vi "spike_data_packete_1.vi"(8 "Log File in":refnum<k34>, 11 "data out":string) -> (3 "output cluster":T1)   [LabVIEW 2017]
uses:
  UI Error Handlers/support/Logging/Control 2.ctl
  Globals/Global - Configuration Options.vi
panel:
  out "data":string
  out "error out":errorcluster
  out "BR3_3 (bending X) 4":i16
  out "data  2":string
  out "SYNC 2":string
  out "BR3_4 (bending X) 4":i16
  out "BR2_4 (torsion) 4":i16
  out "BR1_4 (axial_force_ 4":i16
  out "BR4_7 (bending Y) 7":i16
  out "BR3_7 (bending X) 7":i16
  out "BR2_7 (torsion)6 2":i16
  out "BR1_7 (axial_force_ 7":i16
  out "BR4_6 (bending Y) 6":i16
  out "BR3_6 (bending X) 6":i16
  out "BR2_6 (torsion)6":i16
  out "BR1_6 (axial_force_ 6":i16
  out "BR4_5 (bending Y) 5":i16
  out "BR3_5 (bending X) 5":i16
  out "BR2_5 (torsion) 5":i16
  out "BR1_5 (axial_force_ 5":i16
  out "BR4_4 (bending Y) 4":i16
  out "BR4_3 (bending Y) 3":i16
  out "BR2_3 (torsion) 3":i16
  out "BR1_3 (axial_force_ 3":i16
  out "BR4_2 (bending Y) 2":i16
  out "BR3_2 (bending X) 2":i16
  out "BR2_2 (torsion) 2":i16
  out "BR1_2 (axial_force_ 2":i16
  out "BR4_1 (bending Y)":i16
  out "BR3_1 (bending X)":i16
  out "BR2_1 (torsion)":i16
  out "BR1_1 (axial_force)":i16
  out "SPER":i16
  out "SPEF":i8
  out "RSSI":i16
  out "PKT":i16
  out "DIN":i8
  out "CMD":i8
  out "DEV":i8
  out "RES":i8
  out "LEN":i8
  out "SYN":i16
  in  "?":T1
  out "DIN":string
  out "DEV":string
  out "RES":string
  out "LEN":string
  out "SYNC":string
  out "CMD":string
  out "Received Data 4":dbl[](graph)
  out "BR4_5 (bending Y) 5":string
  out "BR3_5 (bending X) 5":string
  out "BR4_7 (bending Y) 7":string
  out "BR3_7 (bending X) 7":string
  out "BR2_7 (torsion)6 2":string
  out "BR1_7 (axial_force_ 7":string
  out "BR4_6 (bending Y) 6":string
  out "BR3_6 (bending X) 6":string
  out "BR2_6 (torsion)6":string
  out "BR1_6 (axial_force_ 6":string
  out "BR2_5 (torsion) 5":string
  out "BR1_5 (axial_force_ 5":string
  out "BR4_4 (bending Y) 4":string
  out "BR3_4 (bending X) 4":string
  out "BR2_4 (torsion) 4":string
  out "BR1_4 (axial_force_ 4":string
  out "BR4_3 (bending Y) 3":string
  out "BR3_3 (bending X) 3":string
  out "BR2_3 (torsion) 3":string
  out "BR1_3 (axial_force_ 3":string
  out "BR4_2 (bending Y) 2":string
  out "BR3_2 (bending X) 2":string
  out "RSSI":string
  out "PKT":string
  out "SPEF":string
  out "SPER":string
  out "BR2_2 (torsion) 2":string
  out "BR1_2 (axial_force_ 2":string
  out "BR4_1 (bending Y)":string
  out "BR3_1 (bending X)":string
  out "BR2_1 (torsion)":string
  out "BR1_1 (axial_force_":string
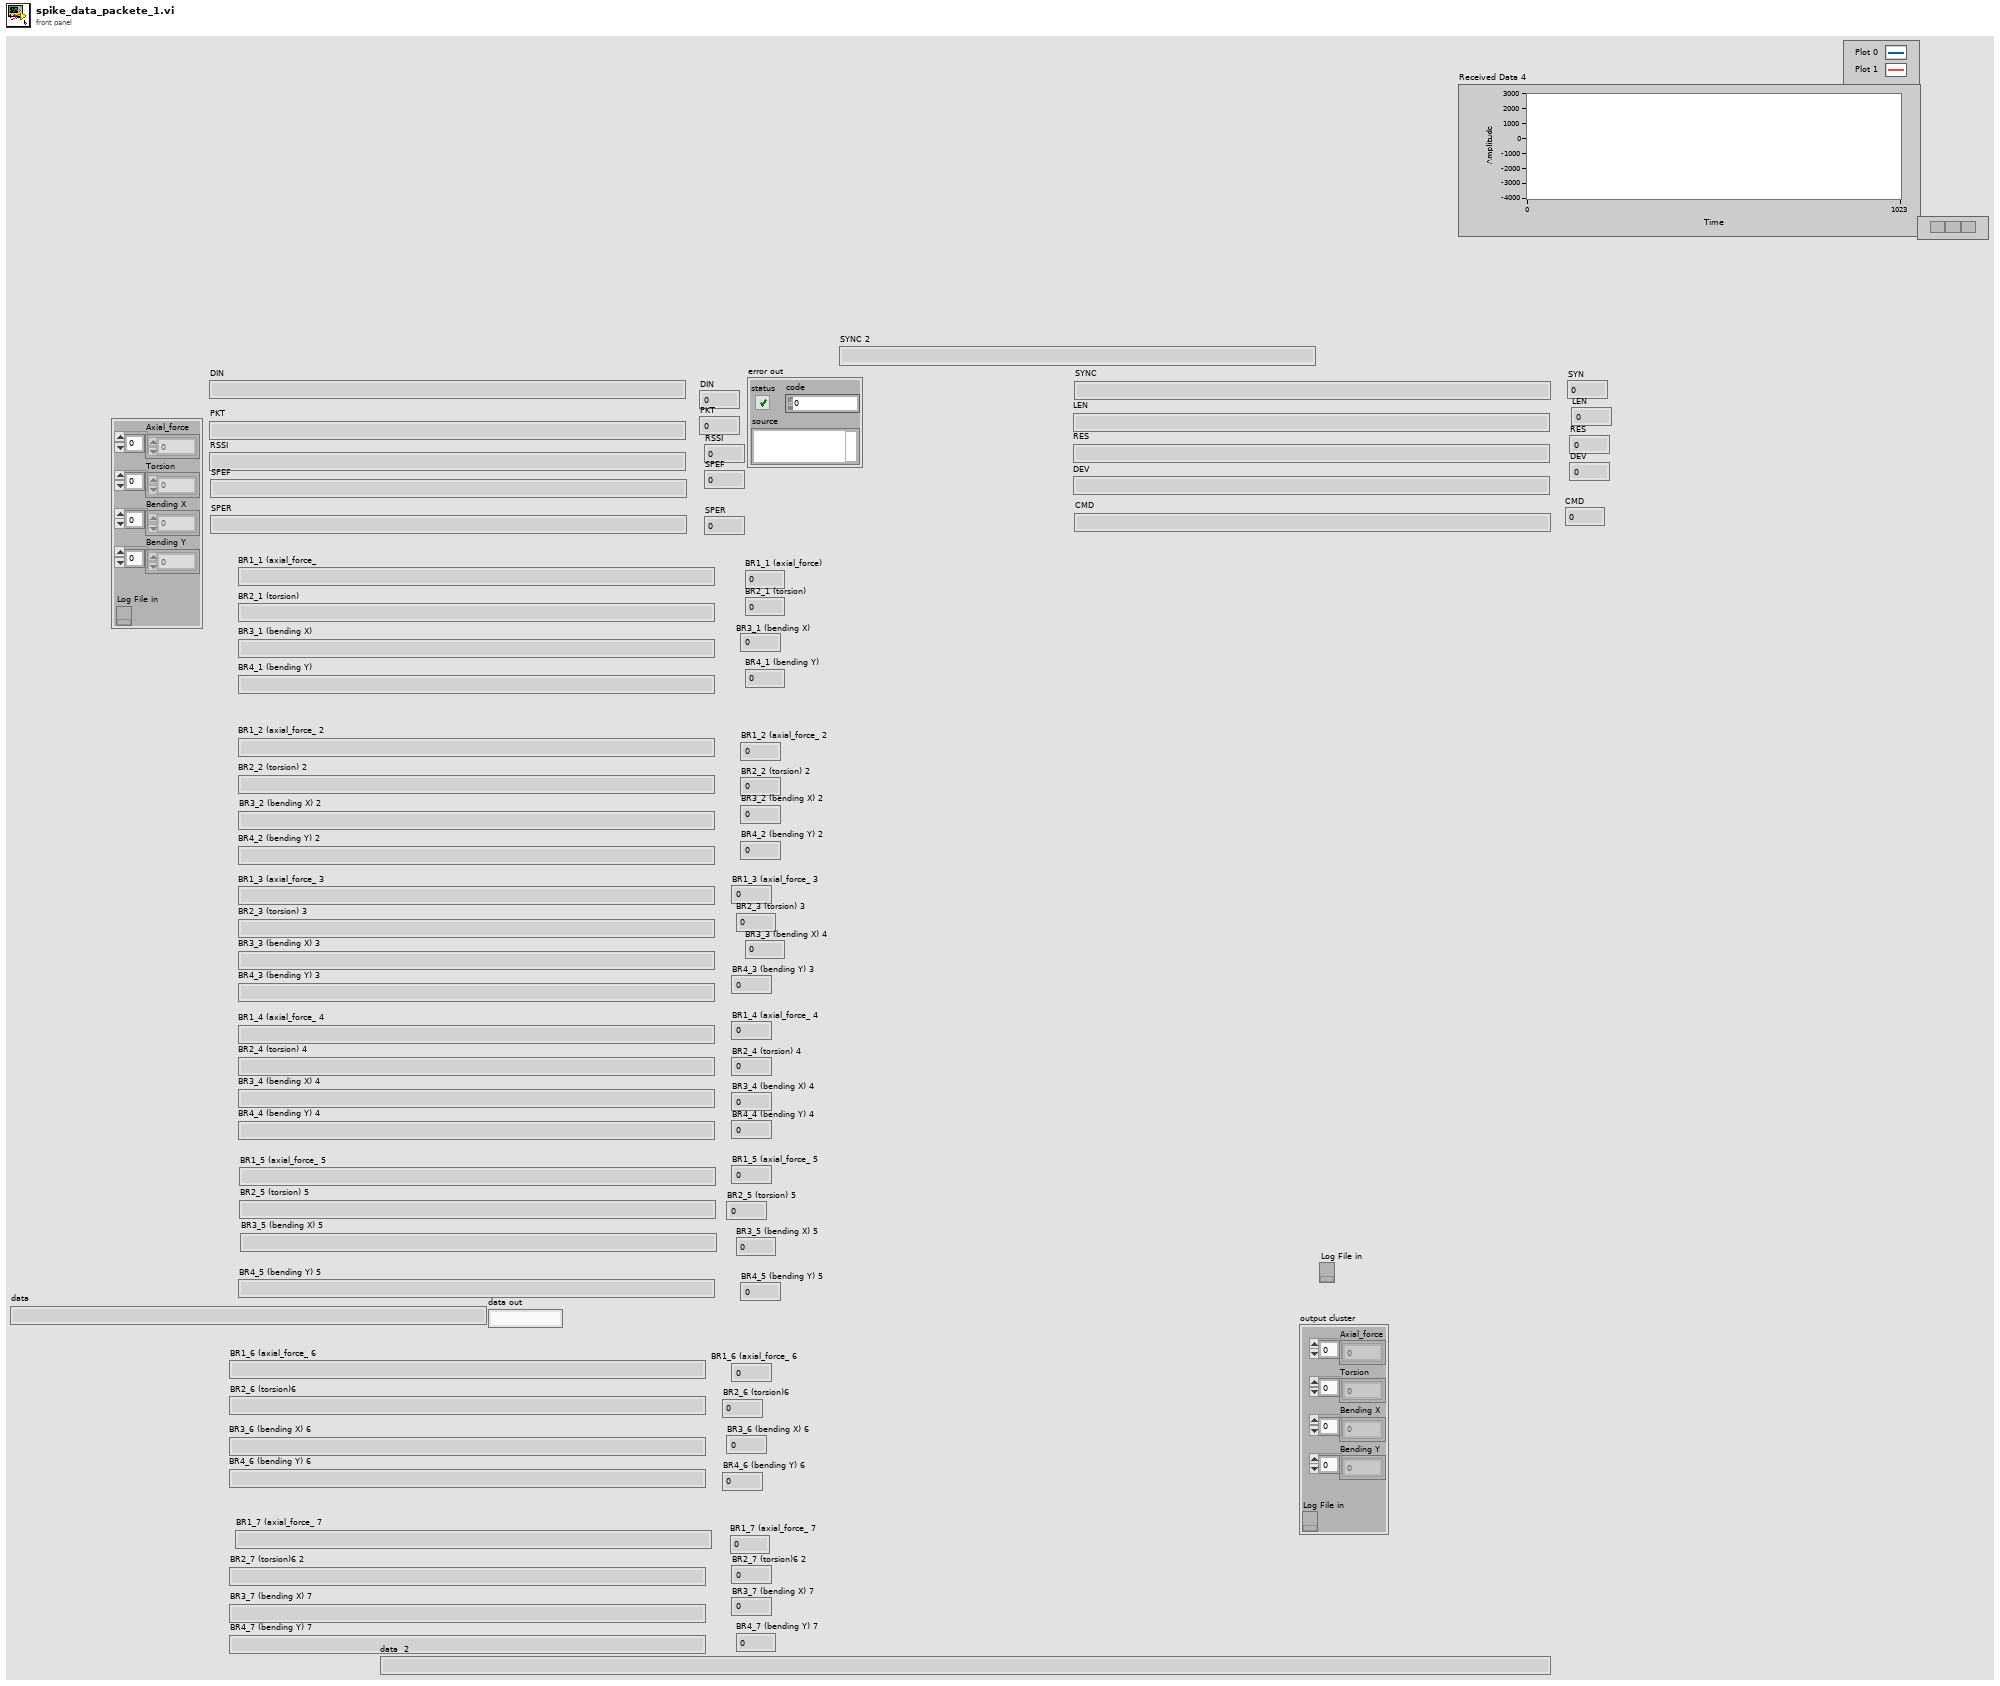
[diagram p1: front panel]
types:
  T1 = typedef "Control 2.ctl" = cluster{"Axial_force":i16[], "Torsion":i16[], "Bending X":i16[], "Bending Y":i16[], "Log File in":refnum<k34>}
  T2 = cluster{"A(I16) 11":i16, "A(I16) 12":i16, "A(I16) 13":i16}
  T3 = cluster{"A(I16) 11":i16, "A(I16) 12":i16, "A(I16) 13":i16, "A(I16) 14":i16, "A(I16) 15":i16, "A(I16) 16":i16, "A(I16) 17":i16}
  T4 = enum16{"big-endian, network order", "native, host order", "little-endian"}
  T5 = cluster{"A(I16)":i16, "A(I8) 2":i8, "A(I8) 3":i8, "A(I18) 4":i8, "A(I8) 5":i8, "A(I8) 6":i8, "A(I16) 7":i16, "A(I8) 8":i8, "A(I8) 9":i8, "A(I16) 10":i16, "A(I16) 11":i16, "A(I16) 12":i16, "A(I16) 13":i16, "A(I16) 14":i16, "A(I16) 15":i16, "A(I16) 16":i16, "A(I16) 17":i16, "A(I16) 18":i16, "A(I16) 19":i16, "A(I16) 20":i16, "A(I16) 21":i16, "A(I16) 22":i16, "A(I16) 23":i16, "A(I16) 24":i16, "A(I16) 25":i16, "A(I16) 26":i16, "A(I16) 27":i16, "A(I16) 28":i16, "A(I16) 29":i16, "A(I16) 30":i16, "A(I16) 31":i16, "A(I16) 32":i16, "A(I16) 33":i16, "A(I16) 34":i16, "A(I16) 35":i16, "A(I16) 36":i16, "A(I16) 37":i16, "A(I16) 38":i16, "A(I16) 39":i16, "A(I16) 40":i16, "A(I16) 41":i16, "A(I16) 42":i16, "A(I16) 43":i16, "A(I16) 44":i16, "A(I16) 45":i16, "A(I16) 46":i16, "A(I16) 47":i16, "A(I16) 48":i16, "A(I16) 49":i16, "A(I16) 50":i16, "A(I16) 51":i16, "A(I16) 52":i16, "A(I16) 53":i16, "A(I16) 54":i16, "A(I16) 55":i16, "A(I16) 56":i16, "A(I16) 57":i16, "A(I16) 58":i16, "A(I16) 59":i16, "A(I16) 60":i16, "A(I16) 61":i16, "A(I16) 62":i16, "A(I16) 63":i16, "A(I16) 64":i16, "A(I16) 65":i16, "A(I16) 66":i16, "A(I16) 67":i16, "A(I16) 68":i16, "A(I16) 69":i16, "A(I16) 70":i16}
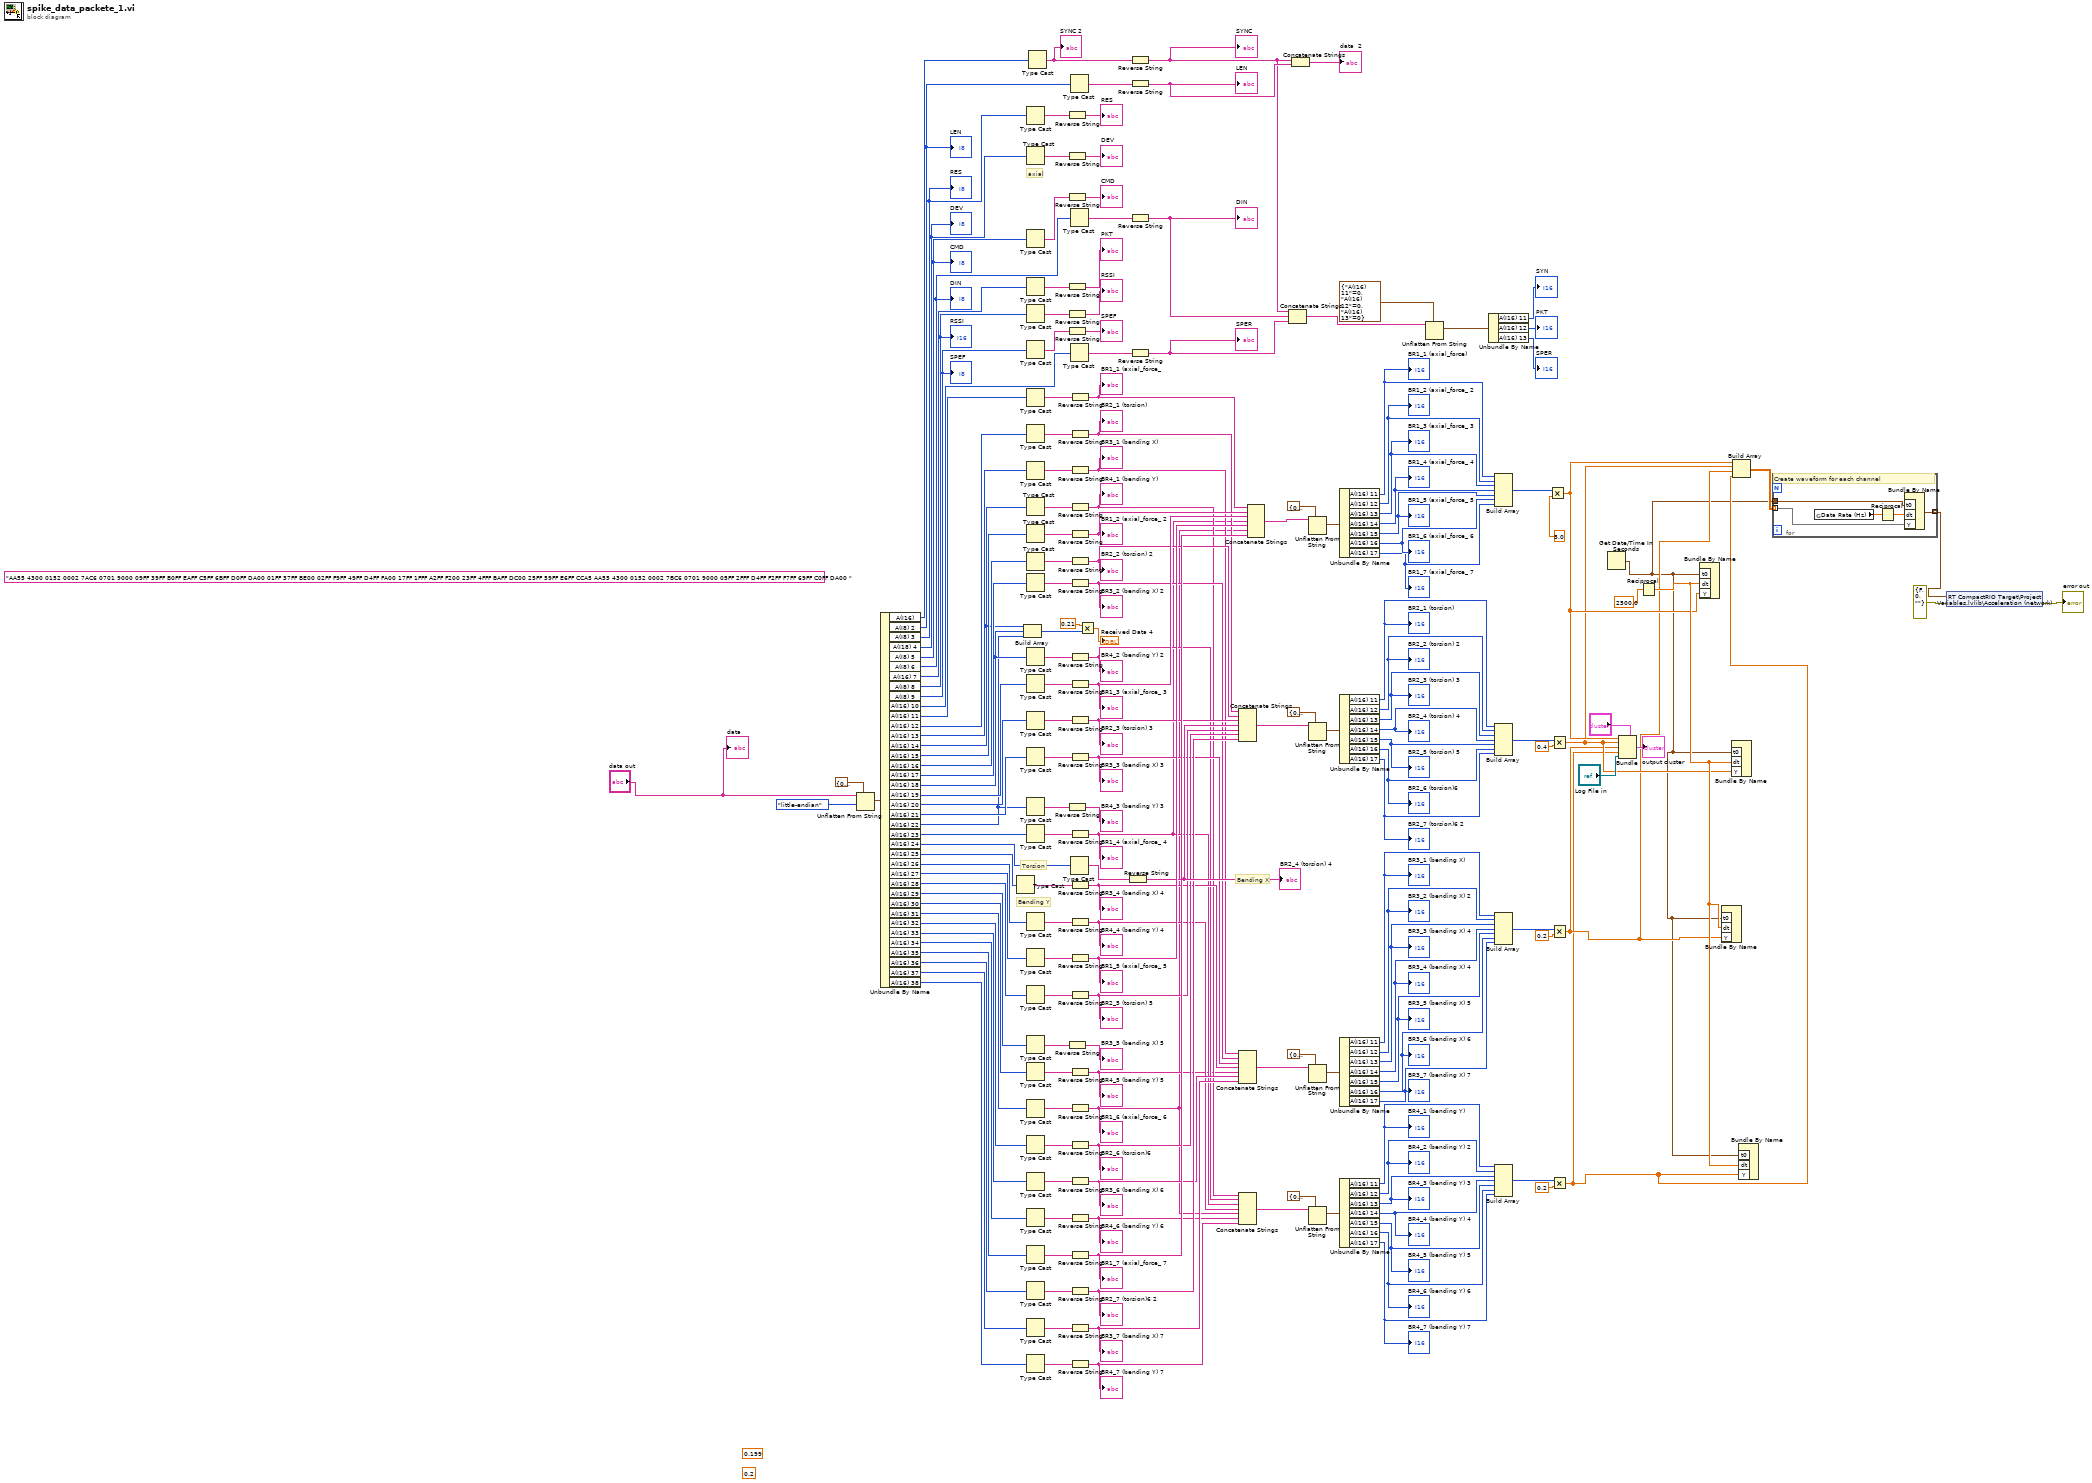
[diagram p0: block diagram]
diagram:
  (unwired) "AA55 4300 0152 0002 7AC6 0701 9000 09FF 39FF B0FF EAFF C5FF 6BFF D0FF DA00 01FF 37FF BE00 02FF F9FF 49FF D4FF FA00 17FF 1FFF A2FF F200 23FF 4FFF BAFF DC00 25FF 59FF E6FF CCA5 AA55 4300 0152 0002 7BC6 0701 9000 05FF 2FFF D4FF F2FF F7FF 69FF C0FF DA00 " ("data")
  (unwired) 0.2
  (unwired) 0.199
  # "Bending Y"
  # "Bending X"
  # "axial"
  # "Torsion"
  n1 = Unflatten From String(type=T5 {"A(I16)"=0, "A(I8) 2"=0, "A(I8) 3"=0, "A(I18) 4"=0, "A(I8) 5"=0, "A(I8) 6"=0, "A(I16) 7"=0, "A(I8) 8"=0, "A(I8) 9"=0, "A(I16) 10"=0, "A(I16) 11"=0, "A(I16) 12"=0, "A(I16) 13"=0, "A(I16) 14"=0, "A(I16) 15"=0, "A(I16) 16"=0, "A(I16) 17"=0, "A(I16) 18"=0, "A(I16) 19"=0, "A(I16) 20"=0, "A(I16) 21"=0, "A(I16) 22"=0, "A(I16) 23"=0, "A(I16) 24"=0, "A(I16) 25"=0, "A(I16) 26"=0, "A(I16) 27"=0, "A(I16) 28"=0, "A(I16) 29"=0, "A(I16) 30"=0, "A(I16) 31"=0, "A(I16) 32"=0, "A(I16) 33"=0, "A(I16) 34"=0, "A(I16) 35"=0, "A(I16) 36"=0, "A(I16) 37"=0, "A(I16) 38"=0, "A(I16) 39"=0, "A(I16) 40"=0, "A(I16) 41"=0, "A(I16) 42"=0, "A(I16) 43"=0, "A(I16) 44"=0, "A(I16) 45"=0, "A(I16) 46"=0, "A(I16) 47"=0, "A(I16) 48"=0, "A(I16) 49"=0, "A(I16) 50"=0, "A(I16) 51"=0, "A(I16) 52"=0, "A(I16) 53"=0, "A(I16) 54"=0, "A(I16) 55"=0, "A(I16) 56"=0, "A(I16) 57"=0, "A(I16) 58"=0, "A(I16) 59"=0, "A(I16) 60"=0, "A(I16) 61"=0, "A(I16) 62"=0, "A(I16) 63"=0, "A(I16) 64"=0, "A(I16) 65"=0, "A(I16) 66"=0, "A(I16) 67"=0, "A(I16) 68"=0, "A(I16) 69"=0, "A(I16) 70"=0}, binary string="data out", byte order (0:big-endian, network order)=T4."little-endian") -> (value=w148:T5)  [unwired: 2 in, 2 out]
  n2 = Unbundle By Name(w148) -> ("A(I16)"=w140:i16, "A(I8) 2"=w139:i8, "A(I8) 3"=w138:i8, "A(I18) 4"=w133:i8, "A(I8) 5"=w132:i8, "A(I8) 6"=w131:i8, "A(I16) 7"=w130:i16, "A(I8) 8"=w129:i8, "A(I8) 9"=w128:i8, "A(I16) 10"=w127:i16, "A(I16) 11"=w101:i16, "A(I16) 12"=w64:i16, "A(I16) 13"=w63:i16, "A(I16) 14"=w104:i16, "A(I16) 15"=w126:i16, "A(I16) 16"=w118:i16, "A(I16) 17"=w114:i16, "A(I16) 18"=w110:i16, "A(I16) 19"=w125:i16, "A(I16) 20"=w120:i16, "A(I16) 21"=w75:i16, "A(I16) 22"=w58:i16, "A(I16) 23"=w124:i16, "A(I16) 24"=w119:i16, "A(I16) 25"=w57:i16, "A(I16) 26"=w109:i16, "A(I16) 27"=w123:i16, "A(I16) 28"=w117:i16, "A(I16) 29"=w113:i16, "A(I16) 30"=w108:i16, "A(I16) 31"=w122:i16, "A(I16) 32"=w115:i16, "A(I16) 33"=w112:i16, "A(I16) 34"=w107:i16, "A(I16) 35"=w121:i16, "A(I16) 36"=w116:i16, "A(I16) 37"=w111:i16, "A(I16) 38"=w106:i16)
  "LEN" <- w139
  "RES" <- w138
  "DEV" <- w133
  "CMD" <- w132
  "DIN" <- w131
  "RSSI" <- w129
  "SPEF" <- w128
  n3 = Type Cast(x=w57) -> (*(type *) &x=w167:string)  [unwired: 1 in]
  n4 = Build Array(w104, w110, w58) -> (w150:i16[])
  n5 = Type Cast(x=w138) -> (*(type *) &x=w146:string)  [unwired: 1 in]
  n6 = Type Cast(x=w133) -> (*(type *) &x=w145:string)  [unwired: 1 in]
  n7 = Type Cast(x=w132) -> (*(type *) &x=w144:string)  [unwired: 1 in]
  n8 = Type Cast(x=w130) -> (*(type *) &x=w188:string)  [unwired: 1 in]
  n9 = Type Cast(x=w129) -> (*(type *) &x=w187:string)  [unwired: 1 in]
  n10 = Type Cast(x=w128) -> (*(type *) &x=w184:string)  [unwired: 1 in]
  n11 = Type Cast(x=w101) -> (*(type *) &x=w186:string)  [unwired: 1 in]
  n12 = Type Cast(x=w64) -> (*(type *) &x=w183:string)  [unwired: 1 in]
  n13 = Type Cast(x=w63) -> (*(type *) &x=w182:string)  [unwired: 1 in]
  n14 = Type Cast(x=w104) -> (*(type *) &x=w181:string)  [unwired: 1 in]
  n15 = Type Cast(x=w126) -> (*(type *) &x=w180:string)  [unwired: 1 in]
  n16 = Type Cast(x=w118) -> (*(type *) &x=w179:string)  [unwired: 1 in]
  n17 = Type Cast(x=w114) -> (*(type *) &x=w174:string)  [unwired: 1 in]
  n18 = Type Cast(x=w110) -> (*(type *) &x=w175:string)  [unwired: 1 in]
  n19 = Type Cast(x=w125) -> (*(type *) &x=w173:string)  [unwired: 1 in]
  n20 = Type Cast(x=w120) -> (*(type *) &x=w172:string)  [unwired: 1 in]
  n21 = Type Cast(x=w75) -> (*(type *) &x=w171:string)  [unwired: 1 in]
  n22 = Type Cast(x=w58) -> (*(type *) &x=w170:string)  [unwired: 1 in]
  n23 = Type Cast(x=w124) -> (*(type *) &x=w165:string)  [unwired: 1 in]
  n24 = Type Cast(x=w109) -> (*(type *) &x=w168:string)  [unwired: 1 in]
  n25 = Type Cast(x=w123) -> (*(type *) &x=w164:string)  [unwired: 1 in]
  n26 = Type Cast(x=w117) -> (*(type *) &x=w163:string)  [unwired: 1 in]
  n27 = Type Cast(x=w113) -> (*(type *) &x=w154:string)  [unwired: 1 in]
  n28 = Type Cast(x=w108) -> (*(type *) &x=w152:string)  [unwired: 1 in]
  n29 = Type Cast(x=w122) -> (*(type *) &x=w162:string)  [unwired: 1 in]
  n30 = Type Cast(x=w115) -> (*(type *) &x=w159:string)  [unwired: 1 in]
  n31 = Type Cast(x=w112) -> (*(type *) &x=w161:string)  [unwired: 1 in]
  n32 = Type Cast(x=w107) -> (*(type *) &x=w160:string)  [unwired: 1 in]
  n33 = Type Cast(x=w121) -> (*(type *) &x=w155:string)  [unwired: 1 in]
  n34 = Type Cast(x=w116) -> (*(type *) &x=w158:string)  [unwired: 1 in]
  n35 = Type Cast(x=w111) -> (*(type *) &x=w156:string)  [unwired: 1 in]
  n36 = Type Cast(x=w106) -> (*(type *) &x=w157:string)  [unwired: 1 in]
  n37 = Type Cast(x=w140) -> (*(type *) &x=w105:string)  [unwired: 1 in]
  "SYNC 2" <- w105
  n38 = Reverse String(1:w146) -> (0:→"RES":string)
  n39 = Reverse String(1:w145) -> (0:→"DEV":string)
  n40 = Reverse String(1:w144) -> (0:→"CMD":string)
  n41 = Reverse String(1:w188) -> (0:→"PKT":string)
  n42 = Reverse String(1:w187) -> (0:→"RSSI":string)
  n43 = Reverse String(1:w184) -> (0:→"SPEF":string)
  n44 = Reverse String(1:w170) -> (0:→"BR4_3 (bending Y) 3":string)
  n45 = Reverse String(1:w154) -> (0:→"BR3_5 (bending X) 5":string)
  n46 = Type Cast(x=w139) -> (*(type *) &x=w147:string)  [unwired: 1 in]
  n47 = Type Cast(x=w131) -> (*(type *) &x=w137:string)  [unwired: 1 in]
  n48 = Type Cast(x=w127) -> (*(type *) &x=w185:string)  [unwired: 1 in]
  n49 = Type Cast(x=w119) -> (*(type *) &x=w166:string)  [unwired: 1 in]
  n50 = Reverse String(1:w186) -> (0:w13:string)
  "BR1_1 (axial_force_" <- w13
  n51 = Reverse String(1:w183) -> (0:w83:string)
  "BR2_1 (torsion)" <- w83
  n52 = Reverse String(1:w182) -> (0:w62:string)
  "BR3_1 (bending X)" <- w62
  n53 = Reverse String(1:w181) -> (0:w39:string)
  "BR4_1 (bending Y)" <- w39
  n54 = Reverse String(1:w180) -> (0:w100:string)
  "BR1_2 (axial_force_ 2" <- w100
  n55 = Reverse String(1:w179) -> (0:w82:string)
  "BR2_2 (torsion) 2" <- w82
  n56 = Reverse String(1:w174) -> (0:w55:string)
  "BR3_2 (bending X) 2" <- w55
  n57 = Reverse String(1:w175) -> (0:w38:string)
  "BR4_2 (bending Y) 2" <- w38
  n58 = Reverse String(1:w173) -> (0:w99:string)
  "BR1_3 (axial_force_ 3" <- w99
  n59 = Reverse String(1:w172) -> (0:w74:string)
  "BR2_3 (torsion) 3" <- w74
  n60 = Reverse String(1:w171) -> (0:w56:string)
  "BR3_3 (bending X) 3" <- w56
  n61 = Reverse String(1:w165) -> (0:w37:string)
  "BR1_4 (axial_force_ 4" <- w37
  n62 = Reverse String(1:w167) -> (0:w54:string)
  "BR3_4 (bending X) 4" <- w54
  n63 = Reverse String(1:w168) -> (0:w36:string)
  "BR4_4 (bending Y) 4" <- w36
  n64 = Reverse String(1:w164) -> (0:w98:string)
  "BR1_5 (axial_force_ 5" <- w98
  n65 = Reverse String(1:w163) -> (0:w80:string)
  "BR2_5 (torsion) 5" <- w80
  n66 = Reverse String(1:w152) -> (0:w35:string)
  "BR4_5 (bending Y) 5" <- w35
  n67 = Reverse String(1:w162) -> (0:w34:string)
  "BR1_6 (axial_force_ 6" <- w34
  n68 = Reverse String(1:w159) -> (0:w79:string)
  "BR2_6 (torsion)6" <- w79
  n69 = Reverse String(1:w161) -> (0:w53:string)
  "BR3_6 (bending X) 6" <- w53
  n70 = Reverse String(1:w160) -> (0:w33:string)
  "BR4_6 (bending Y) 6" <- w33
  n71 = Reverse String(1:w155) -> (0:w97:string)
  "BR1_7 (axial_force_ 7" <- w97
  n72 = Reverse String(1:w158) -> (0:w78:string)
  "BR2_7 (torsion)6 2" <- w78
  n73 = Reverse String(1:w156) -> (0:w52:string)
  "BR3_7 (bending X) 7" <- w52
  n74 = Reverse String(1:w157) -> (0:w32:string)
  "BR4_7 (bending Y) 7" <- w32
  n75 = Multiply(x=0.21, y=w150) -> (x*y=→"Received Data 4":dbl[])
  n76 = Reverse String(1:w166) -> (0:w81:string)
  "BR2_4 (torsion) 4" <- w81
  n77 = Reverse String(1:w105) -> (0:w22:string)
  "SYNC" <- w22
  n78 = Reverse String(1:w147) -> (0:w103:string)
  "LEN" <- w103
  n79 = Reverse String(1:w137) -> (0:w21:string)
  "DIN" <- w21
  n80 = Reverse String(1:w185) -> (0:w20:string)
  "SPER" <- w20
  n81 = Concatenate Strings(w83, w82, w74, w81, w80, w79, w78) -> (w77:string)
  n82 = Concatenate Strings(w62, w55, w56, w54, w35, w53, w52) -> (w61:string)
  n83 = Concatenate Strings(w39, w38, w37, w36, w34, w33, w32) -> (w40:string)
  n84 = Concatenate Strings(w13, w100, w99, w37, w98, w34, w97) -> (w95:string)
  n85 = Concatenate Strings(w22, w21, w20) -> (w18:string)
  n86 = Concatenate Strings(w22, w103) -> (→"data  2":string)
  n87 = Unflatten From String(type=T3 {"A(I16) 11"=0, "A(I16) 12"=0, "A(I16) 13"=0, "A(I16) 14"=0, "A(I16) 15"=0, "A(I16) 16"=0, "A(I16) 17"=0}, binary string=w95) -> (value=w94:T3)  [unwired: 3 in, 2 out]
  n88 = Unflatten From String(type=T3 {"A(I16) 11"=0, "A(I16) 12"=0, "A(I16) 13"=0, "A(I16) 14"=0, "A(I16) 15"=0, "A(I16) 16"=0, "A(I16) 17"=0}, binary string=w77) -> (value=w76:T3)  [unwired: 3 in, 2 out]
  n89 = Unflatten From String(type=T3 {"A(I16) 11"=0, "A(I16) 12"=0, "A(I16) 13"=0, "A(I16) 14"=0, "A(I16) 15"=0, "A(I16) 16"=0, "A(I16) 17"=0}, binary string=w61) -> (value=w59:T3)  [unwired: 3 in, 2 out]
  n90 = Unflatten From String(type=T3 {"A(I16) 11"=0, "A(I16) 12"=0, "A(I16) 13"=0, "A(I16) 14"=0, "A(I16) 15"=0, "A(I16) 16"=0, "A(I16) 17"=0}, binary string=w40) -> (value=w42:T3)  [unwired: 3 in, 2 out]
  n91 = Unbundle By Name(w94) -> ("A(I16) 11"=w91:i16, "A(I16) 12"=w90:i16, "A(I16) 13"=w89:i16, "A(I16) 14"=w88:i16, "A(I16) 15"=w87:i16, "A(I16) 16"=w86:i16, "A(I16) 17"=w85:i16)
  "BR1_1 (axial_force)" <- w91
  "BR1_2 (axial_force_ 2" <- w90
  "BR1_3 (axial_force_ 3" <- w89
  "BR1_5 (axial_force_ 5" <- w87
  "BR1_6 (axial_force_ 6" <- w86
  "BR1_7 (axial_force_ 7" <- w85
  "BR1_4 (axial_force_ 4" <- w88
  n92 = Unbundle By Name(w76) -> ("A(I16) 11"=w73:i16, "A(I16) 12"=w72:i16, "A(I16) 13"=w71:i16, "A(I16) 14"=w70:i16, "A(I16) 15"=w69:i16, "A(I16) 16"=w68:i16, "A(I16) 17"=w67:i16)
  "BR2_1 (torsion)" <- w73
  "BR2_2 (torsion) 2" <- w72
  "BR2_3 (torsion) 3" <- w71
  "BR2_5 (torsion) 5" <- w69
  "BR2_6 (torsion)6" <- w68
  "BR2_7 (torsion)6 2" <- w67
  "BR2_4 (torsion) 4" <- w70
  n93 = Unbundle By Name(w59) -> ("A(I16) 11"=w51:i16, "A(I16) 12"=w50:i16, "A(I16) 13"=w49:i16, "A(I16) 14"=w48:i16, "A(I16) 15"=w47:i16, "A(I16) 16"=w46:i16, "A(I16) 17"=w45:i16)
  "BR3_1 (bending X)" <- w51
  "BR3_2 (bending X) 2" <- w50
  "BR3_5 (bending X) 5" <- w47
  "BR3_6 (bending X) 6" <- w46
  "BR3_7 (bending X) 7" <- w45
  "BR3_4 (bending X) 4" <- w48
  "BR3_3 (bending X) 4" <- w49
  n94 = Unbundle By Name(w42) -> ("A(I16) 11"=w30:i16, "A(I16) 12"=w28:i16, "A(I16) 13"=w29:i16, "A(I16) 14"=w27:i16, "A(I16) 15"=w26:i16, "A(I16) 16"=w25:i16, "A(I16) 17"=w24:i16)
  "BR4_1 (bending Y)" <- w30
  "BR4_2 (bending Y) 2" <- w28
  "BR4_3 (bending Y) 3" <- w29
  "BR4_4 (bending Y) 4" <- w27
  "BR4_5 (bending Y) 5" <- w26
  "BR4_6 (bending Y) 6" <- w25
  "BR4_7 (bending Y) 7" <- w24
  n95 = Unflatten From String(type=T2 {"A(I16) 11"=0, "A(I16) 12"=0, "A(I16) 13"=0}, binary string=w18) -> (value=w17:T2)  [unwired: 3 in, 2 out]
  n96 = Unbundle By Name(w17) -> ("A(I16) 11"=→"SYN":i16, "A(I16) 12"=→"PKT":i16, "A(I16) 13"=→"SPER":i16)
  n97 = Build Array(w91, w90, w89, w88, w87, w86, w85) -> (w92:i16[])
  n98 = Build Array(w73, w72, w71, w70, w69, w68, w67) -> (w66:i16[])
  n99 = Build Array(w51, w50, w49, w48, w47, w46, w45) -> (w43:i16[])
  n100 = Build Array(w30, w28, w29, w27, w26, w25, w24) -> (w23:i16[])
  n101 = Multiply(x=w92, y=5.0) -> (x*y=w10:dbl[])
  n102 = Multiply(x=w66, y=0.4) -> (x*y=w9:dbl[])
  n103 = Multiply(x=w43, y=0.2) -> (x*y=w8:dbl[])
  n104 = Multiply(x=w23, y=0.2) -> (x*y=w7:dbl[])
  n105 = Get Date/Time In Seconds() -> (seconds since 1Jan1904=w5:timestamp)
  n106 = Bundle(cluster="?", "Axial_force"=w10, "Torsion"=w9, "Bending X"=w8, "Bending Y"=w7, "Log File in"="Log File in") -> (→"output cluster":T1)
  n107 = Reciprocal(x=2500.0) -> (1/x=w11:dbl)
  n108 = Bundle By Name("t0"=w5, "dt"=w11, "Y"=w10) -> ()  [unwired: 1 in, 1 out]
  n109 = Bundle By Name("t0"=w5, "dt"=w11, "Y"=w8) -> ()  [unwired: 1 in, 1 out]
  n110 = Bundle By Name("t0"=w5, "dt"=w11, "Y"=w9) -> ()  [unwired: 1 in, 1 out]
  n111 = Build Array(w10, w9, w8, w7) -> (w6:dbl[][])
  n112 = Bundle By Name("t0"=w5, "dt"=w11, "Y"=w7) -> ()  [unwired: 1 in, 1 out]
  n113 = for {
    tunnel: w6 -> [w195] mode=indexing
    tunnel: w5 -> [w194]
    tunnel: [w192] -> w4 mode=indexing
    # "Create waveform for each channel"
    n114 = global read "Global - Configuration Options.vi" "Data Rate (Hz)"() -> (w191:dbl)
    n115 = Reciprocal(x=w191) -> (1/x=w193:dbl)
    n116 = Bundle By Name("t0"=w194, "dt"=w193, "Y"=w195) -> (w192:waveform(dbl))  [unwired: 1 in]
  }
  n117 = shared-variable "RT CompactRIO Target\\Project Variables.lvlib\\Acceleration (network)"(w4, error in=errorcluster {"status"=FALSE, "code"=0, "source"=""} ("error in (no error)")) -> (error out=→"error out":errorcluster)
  "data" <- "data out"
